vi "Launcher.vi"() -> ()   [LabVIEW 2018, in "EMS Launcher.lvlib"]
doc: "Launcher for the Master Controller SCADA program."
uses:
  EMS Launcher.lvlib
  Global Variables/Controls/Optimization Type Selector.ctl
  EMS User Interface Actor/EMS User Interface/EMS User Interface.lvclass
  C:/Program Files (x86)/National Instruments/LabVIEW 2018/vi.lib/ActorFramework/Actor/Actor.lvclass
  Global Variables/Global Variables.vi
  <vilib>/ActorFramework/Actor/Actor.lvclass
panel:
  in  "Enable Remote Operation":bool
  in  "stop":bool
  in  "Networked?":bool
  in  "Specialized Optimization":T1=enum."Single Phase"
  in  "Per-Unitize?":bool
  # "This is the top launcher of the EMS application. After running this a seperate window will open that provides the interface to the EMS."
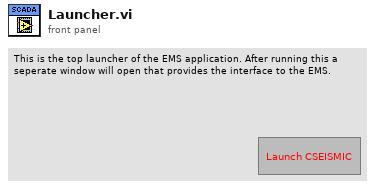
[diagram p1: front panel]
types:
  T1 = typedef "Optimization Type Selector.ctl" = enum16{"Invalid", "Single Phase", "Volttron"}
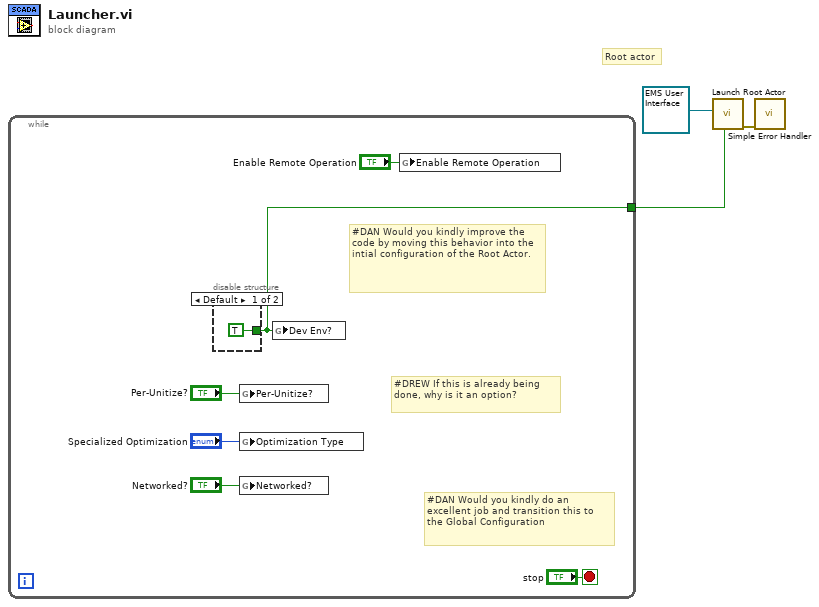
[diagram p0: block diagram]
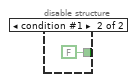
[diagram p2: hidden frame]
diagram:
  # "Root actor"
  n1 = while {
    tunnel: [w9] -> w1
    stop <- "stop" stop-if-true
    # "#DAN Would you kindly do an excellent job and transition this to the Global Configuration"
    # "#DREW If this is already being done, why is it an option?"
    # "#DAN Would you kindly improve the code by moving this behavior into the intial configuration of the Root Actor."
    n2 = disable-structure shown="Default" {
      disable-tunnel: [TRUE ("Dev Env?") FALSE] -> w9
      frame condition #0 (active) {
      }
      frame condition #1 {
      }
    }
    n3 = global write "Global Variables.vi" "Per-Unitize?"("Per-Unitize?") -> ()
    n4 = global write "Global Variables.vi" "Optimization Type"("Specialized Optimization") -> ()
    n5 = global write "Global Variables.vi" "Networked?"("Networked?") -> ()
    n6 = global write "Global Variables.vi" "Dev Env?"(w9) -> ()
    n7 = global write "Global Variables.vi" "Enable Remote Operation"("Enable Remote Operation") -> ()
  }
  n8 = call <vilib>:"Launch Root Actor.vi"("Open Actor Core front panel? (F)"=w1, "Actor"=refnum<class "EMS User Interface.lvclass"> refnum ("Master Controller Core.lvlib:Master Controller.lvclass")) -> ("error out"=w3:errorcluster)  [unwired: 8 in, 1 out]
  n9 = call <vilib>:"Simple Error Handler.vi"("error in (no error)"=w3) -> ()  [unwired: 4 in, 5 out]
